vi "BLE_Get_WatcherReceivedData.vi"(0 ".NET Refnum in":refnum<k24>, 11 "error in (no error)":errorcluster) -> (3 "M_Data":string[](array[string]), 4 ".NET Refnum out":refnum<k24>, 6 "Watcher Response":string, 8 "Bluetooth Addr":string[](array[string]), 10 "Bluetooth Raw Addr":string[](array[string]), 13 "RSSI":string[](array[string]), 14 "Manf_ID":string[](array[string]), 15 "error out":errorcluster)   [LabVIEW 2020]
uses:
  C:/Users/bharathi.t/Downloads/Bluetooth - Copy/Bluetooth/BLE/BLELib.dll
  BLELib.dll
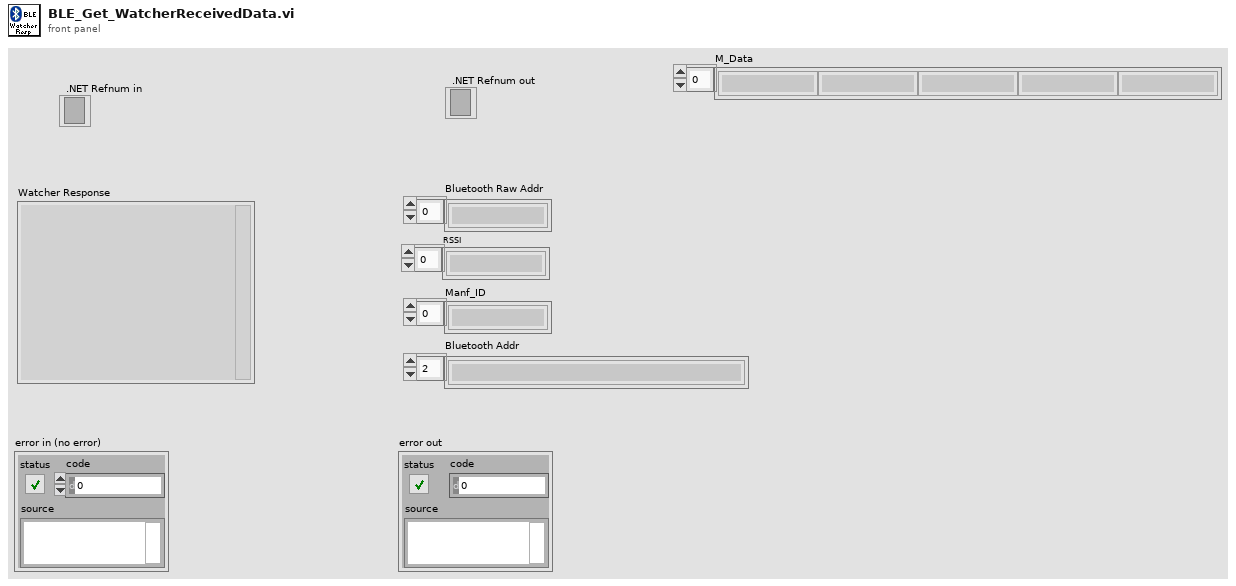
[diagram p1: front panel]
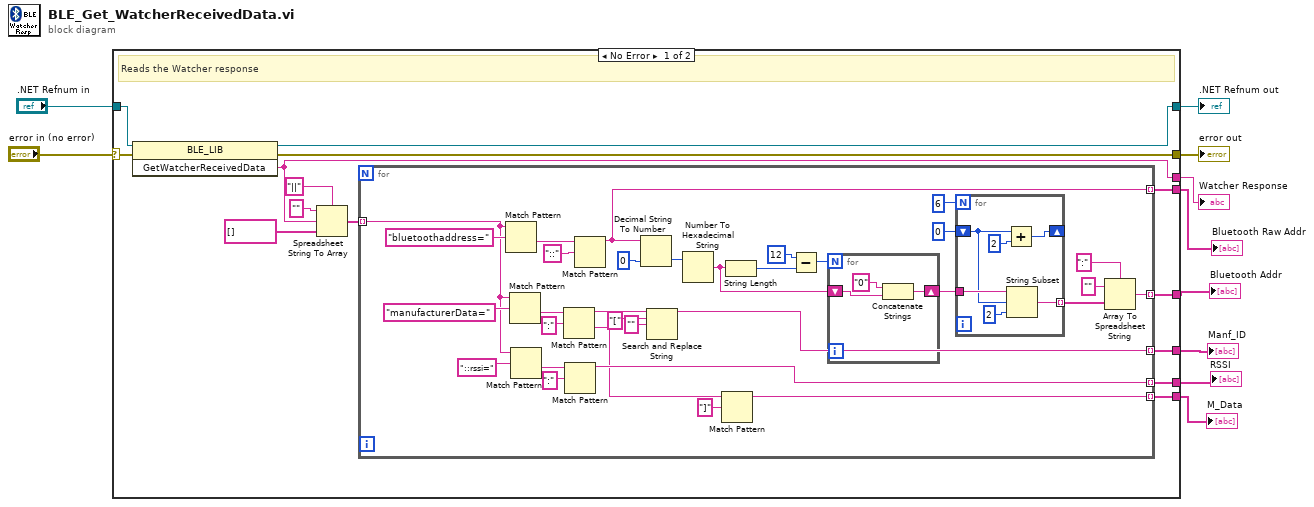
[diagram p0: block diagram]
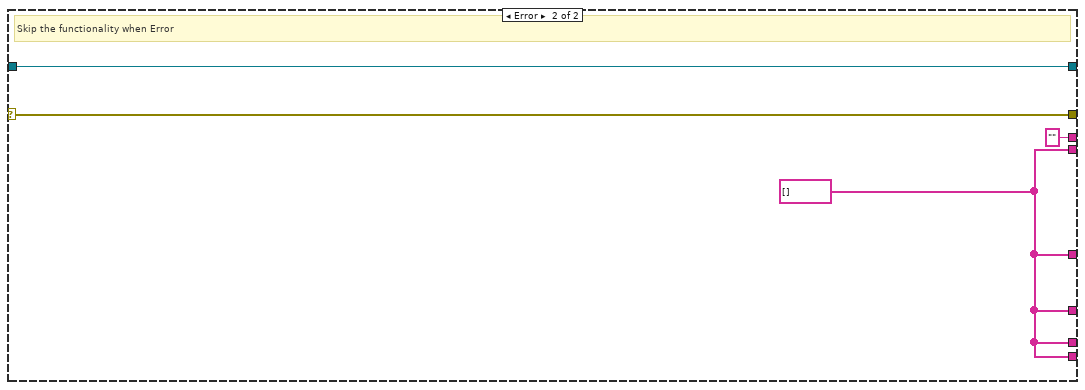
[diagram p2: hidden frame]
diagram:
  n1 = case shown="No Error" "error in (no error)" {
    selector: "error in (no error)" -> [w21 w68]
    tunnel: ".NET Refnum in" -> [w24 w69]
    tunnel: [w23 w68] -> w9
    tunnel: [w22 w69] -> w8
    tunnel: [w14 "" ("GetWatcherReceivedData")] -> w6
    tunnel: [w19 w66] -> w5
    tunnel: [w20 w66] -> w4
    tunnel: [w13 w66] -> w3
    tunnel: [w12 w66] -> w2
    tunnel: [w11 w66] -> w1
    frame No Error {
      # "Reads the Watcher response"
      n2 = invoke class="BLE_LIB" method="GetWatcherReceivedData"(reference=w24, error in=w21) -> (reference out=w22:refnum<k24>, error out=w23:errorcluster, "GetWatcherReceivedData"=w14:string)  [unwired: 1 in]
      n3 = Spreadsheet String To Array(delimiter (Tab)="||", format string="", spreadsheet string=w14, array type (2D Dbl)=string[] []) -> (array=w15:string[])
      n4 = for {
        tunnel: [w42] -> w20 mode=indexing
        tunnel: [w41] -> w19 mode=indexing
        tunnel: w15 -> [w31] mode=indexing
        tunnel: [w36] -> w13 mode=indexing
        tunnel: [w29] -> w12 mode=indexing
        tunnel: [w25] -> w11 mode=indexing
        n5 = Match Pattern(string=w31, regular expression="bluetoothaddress=") -> (after substring=w52:string)  [unwired: 1 in, 3 out]
        n6 = Match Pattern(string=w31, regular expression="manufacturerData=") -> (after substring=w37:string)  [unwired: 1 in, 3 out]
        n7 = Match Pattern(string=w31, regular expression="::rssi=") -> (after substring=w33:string)  [unwired: 1 in, 3 out]
        n8 = Match Pattern(string=w37, regular expression=":") -> (before substring=w28:string, after substring=w27:string)  [unwired: 1 in, 2 out]
        n9 = Match Pattern(string=w33, regular expression=":") -> (before substring=w29:string)  [unwired: 1 in, 3 out]
        n10 = Match Pattern(string=w52, regular expression="::") -> (before substring=w42:string)  [unwired: 1 in, 3 out]
        n11 = Decimal String To Number(string=w42, default (0L)=i64 0 ("default (0 I32)")) -> (number=w55:i64)  [unwired: 1 in, 1 out]
        n12 = Search and Replace String(input string=w28, search string="[" ("replace string (\"\")"), replace string="" ("replace string (\"\")")) -> (result string=w36:string)  [unwired: 5 in, 3 out]
        n13 = Number To Hexadecimal String(2:w55) -> (0:w48:string)  [unwired: 1 in]
        n14 = Match Pattern(string=w27, regular expression="]") -> (before substring=w25:string)  [unwired: 1 in, 3 out]
        n15 = String Length(string=w48) -> (length=w51:i32)
        n16 = Subtract(x=12, y=w51) -> (x-y=w49:i32)
        n17 = for {
          N: w49 -> [_]
          shift-right: [w63] -> w46
          shift-left: w48 -> [w65]
          n18 = Concatenate Strings("0" ("string"), w65) -> (w63:string)
        }
        n19 = for {
          N: 6 -> [_]
          tunnel: w46 -> [w62]
          shift-right: [w58] -> _
          shift-left: 0 ("offset (0)") -> [w60]
          tunnel: [w57] -> w44 mode=indexing
          n20 = Add(x=w60, y=2) -> (x+y=w58:i32)
          n21 = String Subset(string=w62, offset (0)=w60, length (rest)=2 ("length (rest)")) -> (substring=w57:string)
        }
        n22 = Array To Spreadsheet String(delimiter (Tab)=":", array=w44, 3:"" ("format string")) -> (spreadsheet string=w41:string)
      }
    }
    frame Error {
      w66 = string[] []
      # "Skip the functionality when Error"
    }
  }
  "Watcher Response" <- w6
  "error out" <- w9
  ".NET Refnum out" <- w8
  "Bluetooth Addr" <- w5
  "Bluetooth Raw Addr" <- w4
  "Manf_ID" <- w3
  "RSSI" <- w2
  "M_Data" <- w1
